vi "Show Data Viewer N Plots.vi"(7 "Caption.Text":string, 11 "Graph":cluster{"X":sgl[], "Y":sgl[]}[](graph) caption="Spectrum") -> ()   [LabVIEW 2015]
uses:
  <vilib>/printing/EasyPrintingControls.llb/layout_options.ctl
  <vilib>/printing/EasyPrintingControls.llb/orientation.ctl
  <vilib>/printing/EasyPrintingControls.llb/panel_scaling_for_page.ctl
  <vilib>/printing/EasyPrintingControls.llb/margins.ctl
  <vilib>/printing/EasyPrintingControls.llb/margin_values.ctl
  <vilib>/printing/EasyPrintingControls.llb/measurement_system.ctl
  <vilib>/printing/EasyPrintingControls.llb/printer_options.ctl
  <vilib>/printing/EasyPrintingControls.llb/printing_method.ctl
  <vilib>/printing/EasyPrintingControls.llb/color_or_monochrome.ctl
  <vilib>/printing/EasyPrintingControls.llb/page_header_options.ctl
  <vilib>/printing/EasyPrintingControls.llb/page_headers.ctl
  <vilib>/printing/EasyPrintingControls.llb/page_header_content_options.ctl
  <vilib>/printing/EasyPrinting.llb/Easy Print VI Panel or Documentation (path).vi
  <vilib>/Utility/NIReport.llb/NI_ReportGenerationCore.lvlib
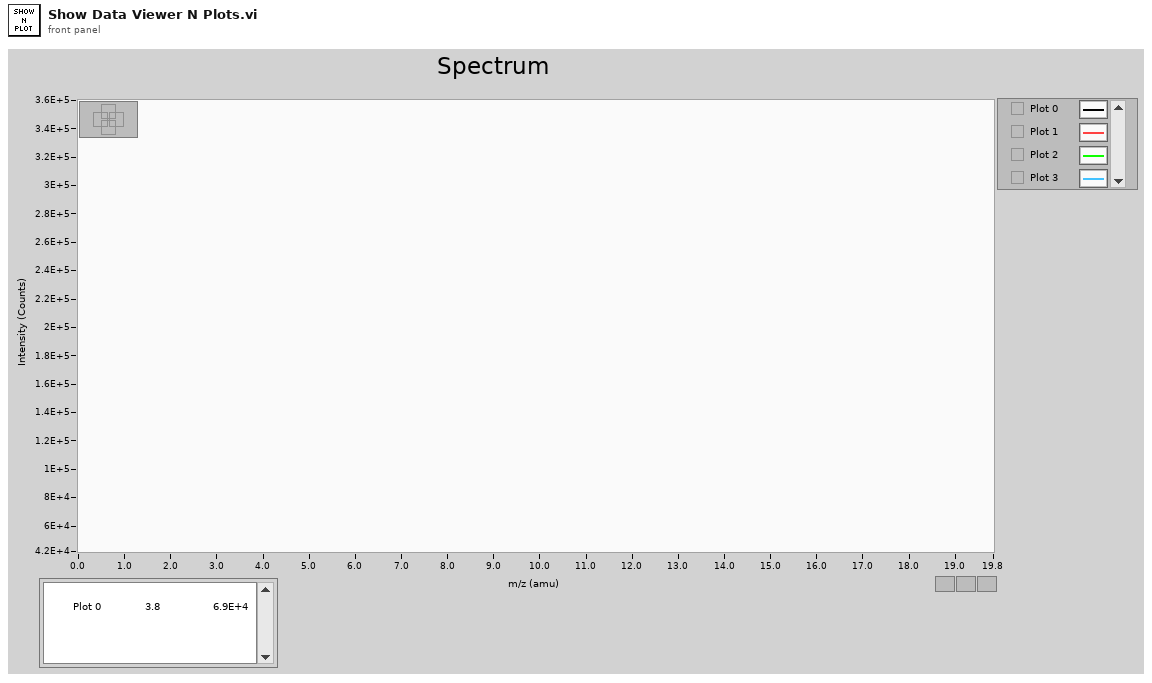
[diagram p1: front panel]
types:
  T1 = typedef "NI_ReportGenerationCore.lvlib/layout_options.ctl" = cluster{"orientation (unchanged)":T2, "panel scaling for page (unchanged)":T3, "margins":T4, "printer options":T7, "page header options":T10}
  T2 = typedef "NI_ReportGenerationCore.lvlib/orientation.ctl" = u16
  T3 = typedef "NI_ReportGenerationCore.lvlib/panel_scaling_for_page.ctl" = u16
  T4 = typedef "NI_ReportGenerationCore.lvlib/margins.ctl" = cluster{"override VI margins (false)":bool, "margins (1.00)":T5, "measurement system (default)":T6}
  T5 = typedef "NI_ReportGenerationCore.lvlib/margin_values.ctl" = cluster{"top":dbl, "left":dbl, "right":dbl, "bottom":dbl}
  T6 = typedef "NI_ReportGenerationCore.lvlib/measurement_system.ctl" = u16
  T7 = typedef "NI_ReportGenerationCore.lvlib/printer_options.ctl" = cluster{"destination printer name (current)":string, "printing method (unchanged)":T8, "color or monochrome (unchanged)":T9}
  T8 = typedef "NI_ReportGenerationCore.lvlib/printing_method.ctl" = u16
  T9 = typedef "NI_ReportGenerationCore.lvlib/color_or_monochrome.ctl" = u16
  T10 = typedef "NI_ReportGenerationCore.lvlib/page_header_options.ctl" = cluster{"page headers (unchanged)":T11, "page header content options":T12}
  T11 = typedef "NI_ReportGenerationCore.lvlib/page_headers.ctl" = u16
  T12 = typedef "NI_ReportGenerationCore.lvlib/page_header_content_options.ctl" = cluster{"Include VI Name":bool, "Include VI Path":bool, "Include Last Modification Date":bool, "Include Date Printed":bool, "Include Page Number":bool, "Include VI Icon":bool}
  T13 = typedef "imagedata.ctl" = cluster{"image type":i32, "image depth":i32, "image":u8[], "mask":u8[], "colors":u32[], "Rectangle":cluster{"left":i16, "top":i16, "right":i16, "bottom":i16}}
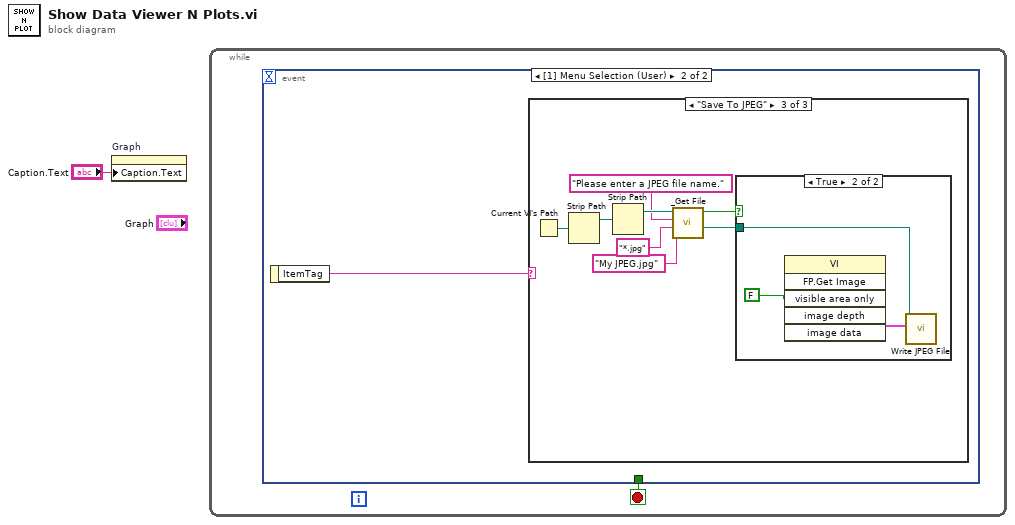
[diagram p0: block diagram]
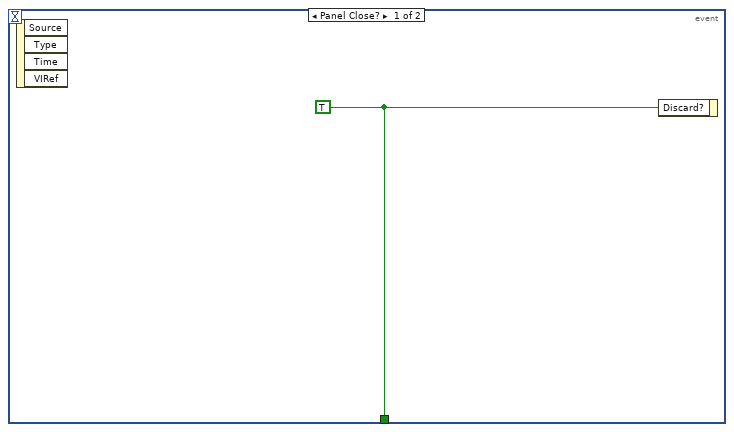
[diagram p2: hidden frame]
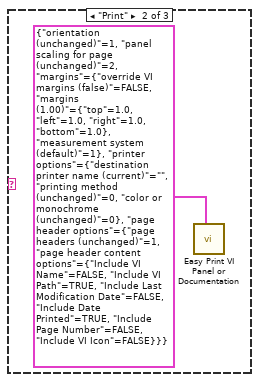
[diagram p4: hidden frame]
diagram:
  n1 = property on="Graph" class="XYGraph (strict)"("Caption.Text"="Caption.Text") -> ()  [unwired: 2 in, 2 out]
  n2 = while {
    stop <- w2 stop-if-true
    n3 = event shown="[1] Menu Selection (User)" {
      selector: _ -> [_ _]
      dyn-events: _ -> [_ _]
      timeout: _ -> [_ _]
      tunnel: [w3 _] -> w2
      event Panel Close? {
        w3 = TRUE ("Discard?")
        n4 = event-data() -> ()  [unwired: 5 out]
        n5 = event-data("Discard?"=w3) -> ()  [unwired: 1 in, 1 out]
      }
      event Menu Selection (User) {
        n6 = event-data() -> ("ItemTag"=w4:string)  [unwired: 1 out]
        n7 = case shown="\"Save To JPEG\"" w4 {
          frame Default {
          }
          frame "Print" {
            n8 = call-poly <vilib>:"Easy Print VI Panel or Documentation.vi"("layout options"=T1 {"orientation (unchanged)"=1, "panel scaling for page (unchanged)"=2, "margins"={"override VI margins (false)"=FALSE, "margins (1.00)"={"top"=1.0, "left"=1.0, "right"=1.0, "bottom"=1.0}, "measurement system (default)"=1}, "printer options"={"destination printer name (current)"="", "printing method (unchanged)"=0, "color or monochrome (unchanged)"=0}, "page header options"={"page headers (unchanged)"=1, "page header content options"={"Include VI Name"=FALSE, "Include VI Path"=TRUE, "Include Last Modification Date"=FALSE, "Include Date Printed"=TRUE, "Include Page Number"=FALSE, "Include VI Icon"=FALSE}}}) -> ()  [unwired: 4 in, 7 out]
          }
          frame "Save To JPEG" {
            n9 = Current VI's Path() -> (path=w13:path)
            n10 = Strip Path(path=w13) -> (stripped path=w12:path)  [unwired: 1 out]
            n11 = Strip Path(path=w12) -> (stripped path=w11:path)  [unwired: 1 out]
            n12 = call "_Get File.vi"("default name"="My JPEG.jpg", "extension (isd)"="*.jpg", "prompt"="Please enter a JPEG file name.", "Start Path"=w11) -> ("Seleted File"=w6:path, "Succeeded"=w7:bool)  [unwired: 2 in, 2 out]
            n13 = case shown="True" w7 {
              tunnel: w6 -> [_ w14]
              frame False {
              }
              frame True {
                n14 = invoke class="VI" method="FP.Get Image"("visible area only"=FALSE ("Visible Area Only")) -> ("image data"=w15:T13)  [unwired: 5 in, 5 out]
                n15 = call <vilib>:"Write JPEG File.vi"("image data"=w15, "path to JPEG file"=w14) -> ()  [unwired: 1 in, 9 out]
              }
            }
          }
        }
      }
    }
  }
